vi "Config_Unidades.vi"() -> ()   [LabVIEW 2015]
uses:
  <vilib>/Analysis/Matrix/Datatypes/RealMatrix.ctl
  <vilib>/Analysis/Matrix/Numeric/Conversions/Matrix To Array - RM.vi
  <vilib>/Analysis/Matrix/NI_Matrix.lvlib
panel:
  out "error out":errorcluster
  out "size(s)":i32
  in  "Ruta del archivo donde se guarda unidades.bin":path=path "Z:/GFERNANDEZ/LABVIEW/WD_NI9233/Configuracion WHD/unidades.bin"
  in  "Unidad     Ejes   Leve Izq   Moder Izq   Grave Izq   Leve Dcha Moder Dcha  Grave Dcha":T1=[[501.0, 16.0, 90.0, 115.0, 130.0, 80.0, 100.0, 130.0], [502.0, 16.0, 90.0, 115.0, 130.0, 80.0, 100.0, 130.0], [503.0, 16.0, 80.0, 100.0, 130.0, 70.0, 90.0, 120.0], [504.0, 16.0, 80.0, 100.0, 130.0, 70.0, 90.0, 120.0], [505.0, 16.0, 80.0, 100.0, 130.0, 70.0, 90.0, 120.0], [506.0, 16.0, 80.0, 100.0, 130.0, 70.0, 90.0, 120.0], [507.0, 16.0, 85.0, 100.0, 130.0, 70.0, 90.0, 120.0], [508.0, 16.0, 80.0, 100.0, 130.0, 70.0, 90.0, 120.0], [509.0, 16.0, 90.0, 115.0, 130.0, 80.0, 100.0, 130.0], [510.0, 16.0, 80.0, 100.0, 130.0, 70.0, 90.0, 120.0], [511.0, 16.0, 85.0, 100.0, 130.0, 70.0, 90.0, 120.0], [512.0, 20.0, 85.0, 100.0, 130.0, 70.0, 90.0, 120.0], [513.0, 20.0, 90.0, 115.0, 130.0, 80.0, 100.0, 130.0], [514.0, 20.0, 90.0, 115.0, 130.0, 80.0, 100.0, 130.0], [515.0, 20.0, 90.0, 100.0, 130.0, 80.0, 100.0, 130.0], [516.0, 20.0, 90.0, 115.0, 130.0, 80.0, 100.0, 130.0], [517.0, 20.0, 90.0, 115.0, 130.0, 80.0, 100.0, 130.0], [518.0, 20.0, 85.0, 100.0, 130.0, 70.0, 90.0, 120.0], [519.0, 20.0, 85.0, 100.0, 130.0, 70.0, 90.0, 120.0], [520.0, 20.0, 80.0, 100.0, 130.0, 70.0, 90.0, 120.0], [521.0, 20.0, 90.0, 115.0, 130.0, 80.0, 100.0, 130.0], [522.0, 20.0, 80.0, 100.0, 130.0, 70.0, 90.0, 120.0], [523.0, 16.0, 80.0, 100.0, 130.0, 70.0, 90.0, 120.0], [524.0, 20.0, 95.0, 115.0, 130.0, 80.0, 100.0, 130.0], [551.0, 16.0, 95.0, 115.0, 130.0, 80.0, 100.0, 130.0], [552.0, 16.0, 95.0, 115.0, 130.0, 80.0, 100.0, 130.0], [553.0, 16.0, 95.0, 115.0, 130.0, 80.0, 100.0, 130.0], [554.0, 16.0, 95.0, 115.0, 130.0, 80.0, 100.0, 130.0], [555.0, 16.0, 95.0, 115.0, 130.0, 80.0, 100.0, 130.0], [556.0, 16.0, 95.0, 115.0, 130.0, 80.0, 100.0, 130.0], [557.0, 16.0, 95.0, 115.0, 130.0, 80.0, 100.0, 130.0], [558.0, 16.0, 95.0, 115.0, 130.0, 80.0, 100.0, 130.0], [559.0, 16.0, 95.0, 115.0, 130.0, 80.0, 100.0, 130.0], [560.0, 16.0, 95.0, 115.0, 130.0, 80.0, 100.0, 130.0], [561.0, 16.0, 95.0, 115.0, 130.0, 80.0, 100.0, 130.0], [562.0, 16.0, 95.0, 115.0, 130.0, 80.0, 100.0, 130.0], [563.0, 16.0, 95.0, 115.0, 130.0, 80.0, 100.0, 130.0], [601.0, 20.0, 95.0, 115.0, 130.0, 80.0, 100.0, 130.0], [602.0, 20.0, 95.0, 115.0, 130.0, 80.0, 100.0, 130.0], [603.0, 20.0, 95.0, 115.0, 130.0, 80.0, 100.0, 130.0], [604.0, 20.0, 95.0, 115.0, 130.0, 80.0, 100.0, 130.0], [605.0, 20.0, 95.0, 115.0, 130.0, 80.0, 100.0, 130.0], [606.0, 20.0, 95.0, 115.0, 130.0, 80.0, 100.0, 130.0], [607.0, 20.0, 95.0, 115.0, 130.0, 80.0, 100.0, 130.0], [608.0, 20.0, 95.0, 115.0, 130.0, 80.0, 100.0, 130.0], [609.0, 20.0, 95.0, 115.0, 130.0, 80.0, 100.0, 130.0], [0.0, 0.0, 16.0, 130.0, 150.0, 80.0, 100.0, 130.0], [888.0, 0.0, 16.0, 130.0, 150.0, 80.0, 100.0, 130.0]]
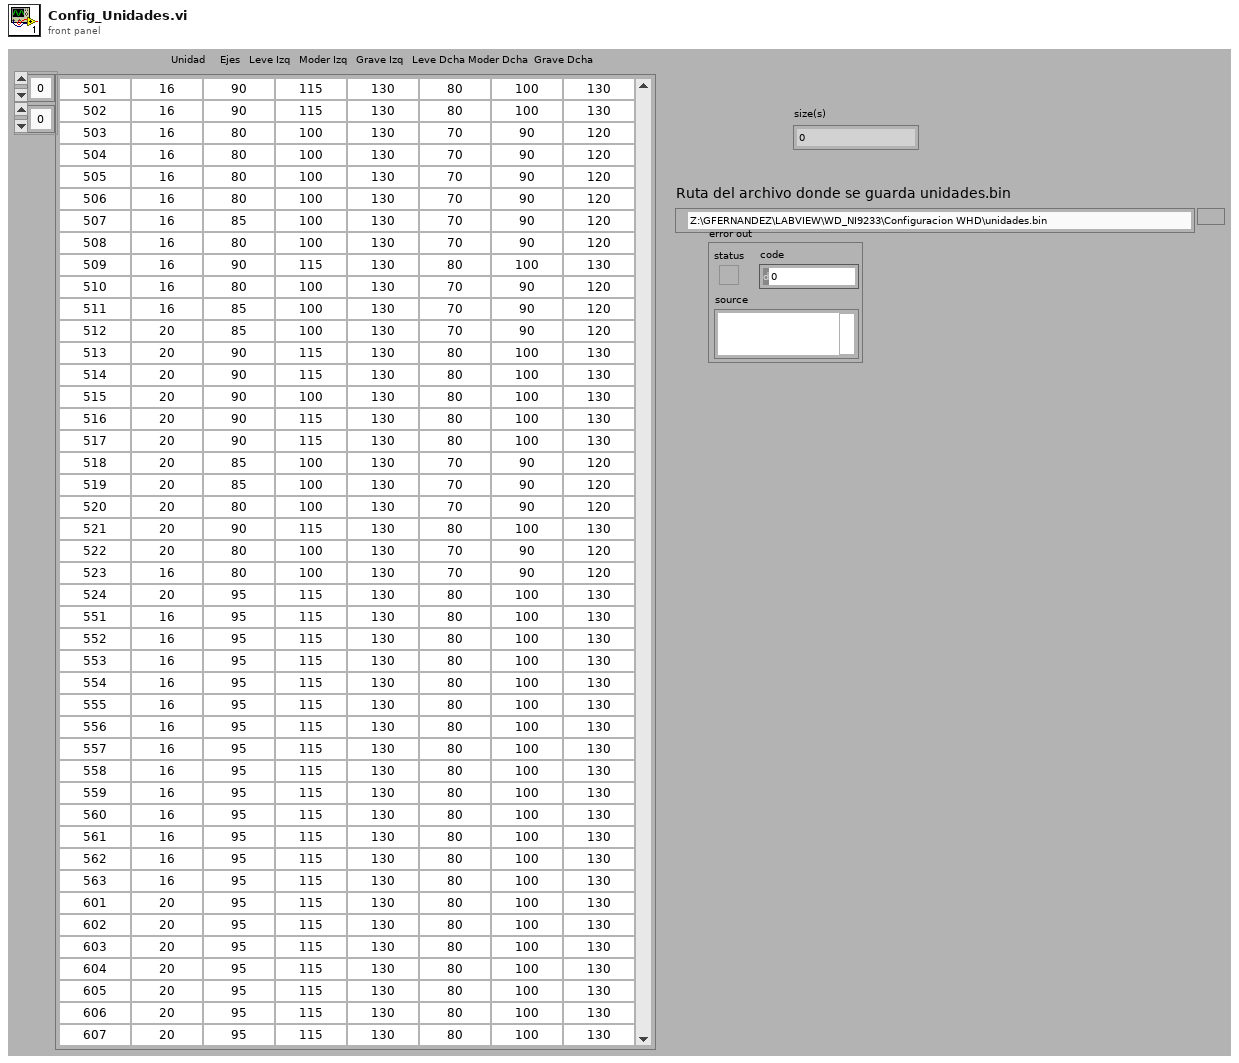
[diagram p1: front panel]
types:
  T1 = typedef "NI_Matrix.lvlib/RealMatrix.ctl" = dbl[][]
  T2 = enum16{"big-endian, network order", "native, host order", "little-endian"}
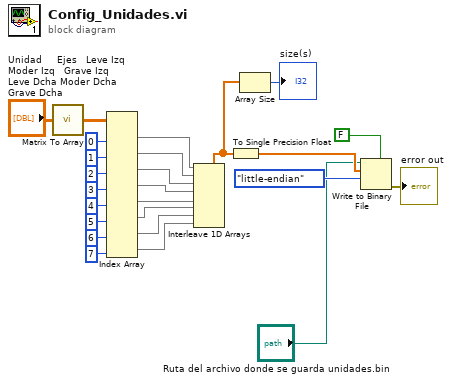
[diagram p0: block diagram]
diagram:
  n1 = call-poly <vilib>:"Matrix To Array.vi"("Real Matrix"="Unidad     Ejes   Leve Izq   Moder Izq   Grave Izq   Leve Dcha Moder Dcha  Grave Dcha") -> ("Real 2D Array"=w24:dbl[][])
  n2 = Index Array(array=w24, index (col) #1=0 ("disabled index (col)"), index (col) #2=1 ("index (col)"), index (col) #3=2 ("index (col)"), index (col) #4=3 ("index (col)"), index (col) #5=4 ("index (col)"), index (col) #6=5 ("index (col)"), index (col) #7=6 ("index (col)"), index (col) #8=7 ("index (col)")) -> (element #1=w20:dbl[], element #2=w21:dbl[], element #3=w6:dbl[], element #4=w5:dbl[], element #5=w4:dbl[], element #6=w3:dbl[], element #7=w2:dbl[], element #8=w1:dbl[])  [unwired: 8 in]
  n3 = Interleave 1D Arrays(w20, w21, w6, w5, w4, w3, w2, w1) -> (w15:dbl[])
  n4 = To Single Precision Float(number=w15) -> (single precision float=w17:sgl[])
  n5 = Array Size(array=w15) -> (size(s)=→"size(s)":i32)
  n6 = Write to Binary File(file (use dialog)="Ruta del archivo donde se guarda unidades.bin", data=w17, 5:FALSE ("prepend array or string size? (T)"), 9:T2."little-endian" ("byte order (0:big-endian, network order)")) -> (error out=→"error out":errorcluster)  [unwired: 1 in, 3 out]
